vi "RunHTTPServer.vi"(0 "Paths":T1={"Root"=path "/Kimberly/Applications/ROBOLAB 2.9/vi.lib/RoboBookEngine/RootFolder", "Shelves"=path "/Kimberly/Users/crogers/Documents/ROBOLAB Data/RoboBooks/Shelves", "Cmds"=path "/Kimberly/Applications/ROBOLAB 2.9/vi.lib/RoboBookEngine/HTTPServer/ServerCommands", "Plugins"=path "/Kimberly/Applications/ROBOLAB 2.9/vi.lib/RoboBookEngine/HTTPServer/ServerCommands"}) -> ()   [LabVIEW 2012]
uses:
  <userlib>/BotSpeak/Devices/EvalRIO/HTTPServer/PathsGlobal.ctl
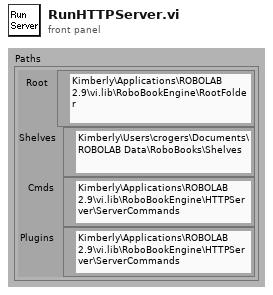
[diagram p1: front panel]
types:
  T1 = typedef "PathsGlobal.ctl" = cluster{"Root":path, "Shelves":path, "Cmds":path, "Plugins":path}
  T2 = enum32{"Bad", "Idle", "Run top level", "Running"}
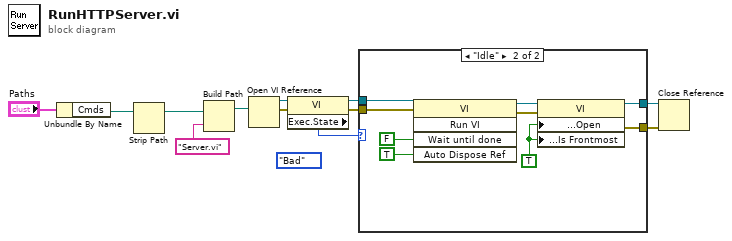
[diagram p0: block diagram]
diagram:
  (unwired) T2."Bad" ("Execution:State")
  n1 = Unbundle By Name("Paths") -> ("Cmds"=w9:path)
  n2 = Strip Path(path=w9) -> (stripped path=w10:path)  [unwired: 1 out]
  n3 = Build Path(base path=w10, name or relative path="Server.vi") -> (appended path=w8:path)
  n4 = Open VI Reference(vi path=w8) -> (vi reference=w5:refnum<vi>, error out=w3:errorcluster)  [unwired: 2 in, 3 out]
  n5 = property class="VI"(reference=w5, error in=w3) -> (reference out=w4:refnum<vi>, error out=w2:errorcluster, "Exec.State"=w1:T2)
  n6 = case shown="\"Idle\"" w1 {
    tunnel: [w13 w18] -> w7
    tunnel: [w14 w17] -> w6
    tunnel: w4 -> [w14 w16]
    tunnel: w2 -> [w13 w15]
    frame "Bad", Default {
    }
    frame "Idle" {
      w19 = TRUE ("Auto Dispose Ref")
      n7 = invoke class="VI" method="Run VI"(reference=w16, error in=w15, "Wait until done"=FALSE, "Auto Dispose Ref"=TRUE) -> (reference out=w20:refnum<vi>, error out=w21:errorcluster)  [unwired: 1 in, 3 out]
      n8 = property class="VI"(reference=w20, error in=w21, "Front Panel Window:Open"=w19, "Front Panel Window:Is Frontmost"=w19) -> (reference out=w17:refnum<vi>, error out=w18:errorcluster)
    }
  }
  n9 = Close Reference(reference=w6, error in (no error)=w7) -> ()  [unwired: 1 out]
